vi "NiezaininicjalizowanyShiftRegister.vi"(3 "Sumowana":dbl) -> (0 "Suma":dbl, 1 "Inkrementowanie":dbl)   [LabVIEW 2024]
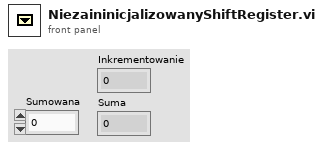
[diagram p1: front panel]
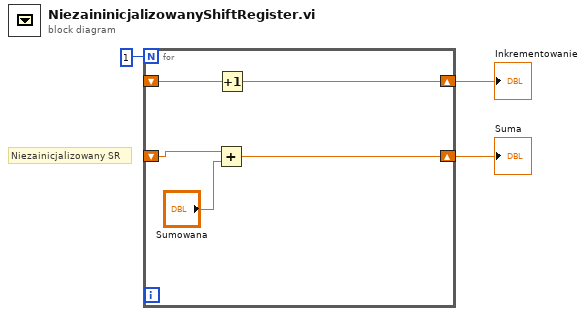
[diagram p0: block diagram]
diagram:
  # "Niezainicjalizowany SR"
  n1 = for {
    N: 1 -> [_]
    shift-right: [w8] -> w2
    shift-left: _ -> [w7]
    shift-right: [w5] -> w1
    shift-left: _ -> [w4]
    n2 = Add(x=w4, y="Sumowana") -> (x+y=w5:dbl)
    n3 = Increment(x=w7) -> (x+1=w8:dbl)
  }
  "Inkrementowanie" <- w2
  "Suma" <- w1
